vi "RSZVB Channel Trace Rename.vi"(8 "error in (no error)":errorcluster {"code" format="%.0x"}, 9 "Trace Name (Trc2)":string="Trc2", 10 "Channel (1)":i32=1, 11 "VISA session":refnum<visa-resource-name>) -> (0 "error out":errorcluster {"code" format="%.0x"}, 3 "dup VISA session":refnum<visa-resource-name>)   [LabVIEW 2011]
doc: "This VI assigns a new name to the active trace in channel <ch>.\n\nRemote-control command(s):\nCONFigure:CHANnel<Ch>TRACe:REName '<trace_name>'"
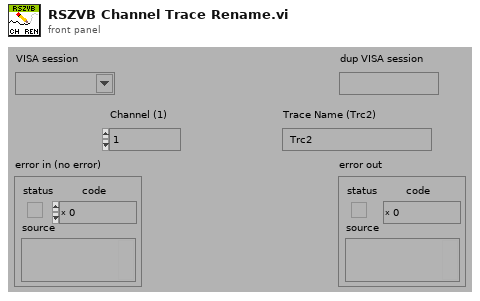
[diagram p1: front panel]
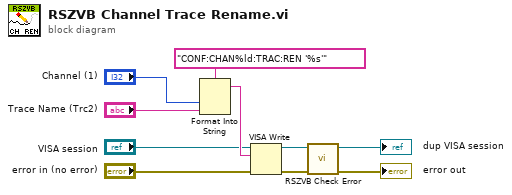
[diagram p0: block diagram]
diagram:
  n1 = Format Into String(format string="CONF:CHAN%ld:TRAC:REN '%s'", "Channel (1)", "Trace Name (Trc2)") -> (resulting string=w7:string)  [unwired: 2 in, 1 out]
  n2 = VISA Write(VISA resource name="VISA session", write buffer=w7, error in (no error)="error in (no error)") -> (VISA resource name out=w8:refnum<visa-resource-name>, error out=w9:errorcluster)  [unwired: 1 out]
  n3 = call "RSZVB Check Error.vi"("error in (no error)"=w9, "VISA session"=w8) -> ("error out"=→"error out":errorcluster, "dup VISA session"=→"dup VISA session":refnum<visa-resource-name>)  [unwired: 8 in]
